vi "manual-move-general.vi"() -> ()   [LabVIEW 2011]
uses:
  <vilib>/userDefined/High Color/IMAQdx.ctl
panel:
  in  "stop":bool
  in  "Ring":u16(ring)=6 items=["*100TW Preamp Up", "*100TW Output Preamp2", "*100TW M0", "*100TW M8", "*100TW M9", "*100TW M10", "*100TW M13", "*100TW M14", "*100TW M20", "*100TW M22", "*100TW M23"]
  out "Names":string[](array[string])=["*100TW Preamp Up", "*100TW Output Preamp2", "*100TW M0", "*100TW M8", "*100TW M9", "*100TW M10", "*100TW M13", "*100TW M14", "*100TW M20", "*100TW M22", "*100TW M23"]
  in  "Step Size":u16=100
  in  "Manual Move":T1={"Down"=FALSE, "Up"=FALSE, "Right"=FALSE, "Left"=FALSE, "APulses X"=200, "APulses Y"=200, "StopButton"=FALSE}
  out "Last Move":string[](array[string])=["", "", "", "", "", "", "3:58:36 PM", "3:59:18 PM", ""]
  in  "CamConfigArray":T3(array[cluster])=[{"ID"=57.0, "Name"="*100TW Preamp Up", "DeviceID"={"Slot Connector"=11, "IP Adress"="192.168.10.34", "Port"=63420, "Type"="picodriver"}, "CorrectConfig Cluster"={"Detection Parameters"={"Contrast"=64, "Treshold"=64, "Max Intensity"=255, "Max Intensity%"=80, "Rx"=95, "Ry"=76, "R%"=70.0}, "Reverse"={"Reverse X"=FALSE, "Reverse Y"=TRUE}, "Target"={"X Target"=387.0, "Y Target"=278.0}, "Region of Interest"=[0, 0, 0, 0], "Correction Parameters"={"X"=30.0, "Y"=30.0, "Movement Type"=1}, "Acquisition Parameters"={"Brightness"=0.0, "Contrast"=0.0, "Saturation"=0.0, "White level"=0.0}, "Background Path"=path "", "Reference Path"=path "", "XCalibration"=[{-240.0, -16.0}, {-210.0, -14.0}, {-180.0, -11.0}, {-150.0, -10.0}, {-120.0, -8.0}, {-90.0, -5.0}, {-60.0, -3.0}, {-30.0, -2.0}, {0.0, -1.0}, {30.0, 0.0}, {60.0, 1.0}, {90.0, 2.0}, {120.0, 5.0}, {150.0, 7.0}, {180.0, 8.0}, {210.0, 9.0}, {240.0, 11.0}, {270.0, 14.0}], "YCalibration"=[{-240.0, 24.0}, {-210.0, 21.0}, {-180.0, 18.0}, {-150.0, 15.0}, {-120.0, 11.0}, {-90.0, 7.0}, {-60.0, 4.0}, {-30.0, 3.0}, {0.0, 1.0}, {30.0, -1.0}, {60.0, -3.0}, {90.0, -4.0}, {120.0, -6.0}, {150.0, -9.0}, {180.0, -12.0}, {210.0, -14.0}, {240.0, -16.0}, {270.0, -18.0}]}, "Ontrak Channel"=0, "IMAQdx Session 2"="cam2", "ImageServer"={"IPAddress"="234.5.6.8", "Port"=58451}}, {"ID"=59.0, "Name"="*100TW Output Preamp2", "DeviceID"={"Slot Connector"=14, "IP Adress"="192.168.10.34", "Port"=63420, "Type"="picodriver"}, "CorrectConfig Cluster"={"Detection Parameters"={"Contrast"=143, "Treshold"=143, "Max Intensity"=255, "Max Intensity%"=80, "Rx"=70, "Ry"=68, "R%"=50.0}, "Reverse"={"Reverse X"=FALSE, "Reverse Y"=FALSE}, "Target"={"X Target"=427.0, "Y Target"=302.0}, "Region of Interest"=[0, 0, 0, 0], "Correction Parameters"={"X"=40.0, "Y"=40.0, "Movement Type"=1}, "Acquisition Parameters"={"Brightness"=0.0, "Contrast"=0.0, "Saturation"=0.0, "White level"=0.0}, "Background Path"=path "", "Reference Path"=path "", "XCalibration"=[{-440.0, -10.0}, {-400.0, -10.0}, {-360.0, -10.0}, {-320.0, -9.0}, {-280.0, -8.0}, {-240.0, -7.0}, {-200.0, -6.0}, {-160.0, -4.0}, {-120.0, -4.0}, {-80.0, -3.0}, {-40.0, -1.0}, {0.0, -1.0}, {40.0, -0.0}, {80.0, 1.0}, {120.0, 2.0}, {160.0, 2.0}, {200.0, 4.0}, {240.0, 5.0}, {280.0, 5.0}, {320.0, 6.0}, {360.0, 7.0}, {400.0, 8.0}, {440.0, 7.0}], "YCalibration"=[{-440.0, 10.0}, {-400.0, 8.0}, {-360.0, 7.0}, {-320.0, 7.0}, {-280.0, 7.0}, {-240.0, 8.0}, {-200.0, 8.0}, {-160.0, 7.0}, {-120.0, 4.0}, {-80.0, 2.0}, {-40.0, 1.0}, {0.0, 1.0}, {40.0, -0.0}, {80.0, -1.0}, {120.0, -2.0}, {160.0, -2.0}, {200.0, -3.0}, {240.0, -3.0}, {280.0, -4.0}, {320.0, -4.0}, {360.0, -4.0}, {400.0, -6.0}, {440.0, -9.0}]}, "Ontrak Channel"=0, "IMAQdx Session 2"="cam2", "ImageServer"={"IPAddress"="234.5.6.8", "Port"=58453}}, {"ID"=60.0, "Name"="*100TW M0", "DeviceID"={"Slot Connector"=13, "IP Adress"="192.168.10.34", "Port"=63420, "Type"="picodriver"}, "CorrectConfig Cluster"={"Detection Parameters"={"Contrast"=58, "Treshold"=58, "Max Intensity"=255, "Max Intensity%"=80, "Rx"=45, "Ry"=42, "R%"=50.0}, "Reverse"={"Reverse X"=FALSE, "Reverse Y"=FALSE}, "Target"={"X Target"=373.0, "Y Target"=310.0}, "Region of Interest"=[0, 0, 0, 0], "Correction Parameters"={"X"=40.0, "Y"=40.0, "Movement Type"=1}, "Acquisition Parameters"={"Brightness"=0.0, "Contrast"=0.0, "Saturation"=0.0, "White level"=0.0}, "Background Path"=path "", "Reference Path"=path "", "XCalibration"=[{-560.0, -7.0}, {-520.0, -7.0}, {-480.0, -7.0}, {-440.0, -7.0}, {-400.0, -6.0}, {-360.0, -5.0}, {-320.0, -4.0}, {-280.0, -4.0}, {-240.0, -4.0}, {-200.0, -3.0}, {-160.0, -2.0}, {-120.0, -2.0}, {-80.0, -1.0}, {-40.0, -0.0}, {0.0, -0.0}, {40.0, -0.0}, {80.0, 0.0}, {120.0, 1.0}, {160.0, 1.0}, {200.0, 2.0}, {240.0, 2.0}, {280.0, 2.0}, {320.0, 2.0}, {360.0, 3.0}, {400.0, 4.0}, {440.0, 5.0}, {480.0, 5.0}, {520.0, 5.0}, {560.0, 5.0}], "YCalibration"=[{-560.0, 3.0}, {-520.0, 3.0}, {-480.0, 3.0}, {-440.0, 3.0}, {-400.0, 3.0}, {-360.0, 4.0}, {-320.0, 3.0}, {-280.0, 3.0}, {-240.0, 3.0}, {-200.0, 2.0}, {-160.0, 1.0}, {-120.0, 1.0}, {-80.0, 0.0}, {-40.0, -0.0}, {0.0, 0.0}, {40.0, 0.0}, {80.0, -0.0}, {120.0, -0.0}, {160.0, -1.0}, {200.0, -2.0}, {240.0, -3.0}, {280.0, -3.0}, {320.0, -3.0}, {360.0, -4.0}, {400.0, -4.0}, {440.0, -4.0}, {480.0, -4.0}, {520.0, -4.0}, {560.0, -4.0}]}, "Ontrak Channel"=0, "IMAQdx Session 2"="cam2", "ImageServer"={"IPAddress"="234.5.6.8", "Port"=58454}}, {"ID"=64.0, "Name"="*100TW M8", "DeviceID"={"Slot Connector"=24, "IP Adress"="192.168.10.34", "Port"=63420, "Type"="picodriver"}, "CorrectConfig Cluster"={"Detection Parameters"={"Contrast"=22, "Treshold"=22, "Max Intensity"=255, "Max Intensity%"=80, "Rx"=225, "Ry"=333, "R%"=50.0}, "Reverse"={"Reverse X"=TRUE, "Reverse Y"=FALSE}, "Target"={"X Target"=731.0, "Y Target"=501.0}, "Region of Interest"=[0, 0, 0, 0], "Correction Parameters"={"X"=50.0, "Y"=50.0, "Movement Type"=1}, "Acquisition Parameters"={"Brightness"=0.0, "Contrast"=0.0, "Saturation"=0.0, "White level"=0.0}, "Background Path"=path "", "Reference Path"=path "", "XCalibration"=[{-450.0, -14.0}, {-400.0, -12.0}, {-350.0, -10.0}, {-300.0, -9.0}, {-250.0, -8.0}, {-200.0, -6.0}, {-150.0, -5.0}, {-100.0, -3.0}, {-50.0, -2.0}, {0.0, -0.0}, {50.0, 1.0}, {100.0, 2.0}, {150.0, 4.0}, {200.0, 6.0}, {250.0, 8.0}, {300.0, 9.0}, {350.0, 11.0}, {400.0, 13.0}, {450.0, 16.0}], "YCalibration"=[{-450.0, 9.0}, {-400.0, 7.0}, {-350.0, 6.0}, {-300.0, 6.0}, {-250.0, 5.0}, {-200.0, 5.0}, {-150.0, 3.0}, {-100.0, 2.0}, {-50.0, 1.0}, {0.0, 0.0}, {50.0, -0.0}, {100.0, -1.0}, {150.0, -3.0}, {200.0, -4.0}, {250.0, -6.0}, {300.0, -7.0}, {350.0, -8.0}, {400.0, -9.0}, {450.0, -11.0}]}, "Ontrak Channel"=0, "IMAQdx Session 2"="cam2", "ImageServer"={"IPAddress"="234.5.6.8", "Port"=58450}}, {"ID"=55.0, "Name"="*100TW M9", "DeviceID"={"Slot Connector"=31, "IP Adress"="192.168.10.34", "Port"=63420, "Type"="picodriver"}, "CorrectConfig Cluster"={"Detection Parameters"={"Contrast"=5, "Treshold"=5, "Max Intensity"=255, "Max Intensity%"=80, "Rx"=400, "Ry"=300, "R%"=50.0}, "Reverse"={"Reverse X"=FALSE, "Reverse Y"=TRUE}, "Target"={"X Target"=771.0, "Y Target"=447.0}, "Region of Interest"=[0, 0, 0, 0], "Correction Parameters"={"X"=40.0, "Y"=40.0, "Movement Type"=1}, "Acquisition Parameters"={"Brightness"=0.0, "Contrast"=0.0, "Saturation"=0.0, "White level"=0.0}, "Background Path"=path "", "Reference Path"=path "", "XCalibration"=[{-320.0, -6.0}, {-280.0, -6.0}, {-240.0, -5.0}, {-200.0, -4.0}, {-160.0, -3.0}, {-120.0, -2.0}, {-80.0, -2.0}, {-40.0, -1.0}, {0.0, -0.0}, {40.0, 0.0}, {80.0, 1.0}, {120.0, 2.0}, {160.0, 2.0}, {200.0, 3.0}, {240.0, 4.0}, {280.0, 4.0}, {320.0, 5.0}, {360.0, 5.0}], "YCalibration"=[{-320.0, 4.0}, {-280.0, 4.0}, {-240.0, 3.0}, {-200.0, 3.0}, {-160.0, 3.0}, {-120.0, 2.0}, {-80.0, 1.0}, {-40.0, 1.0}, {0.0, 0.0}, {40.0, -0.0}, {80.0, -1.0}, {120.0, -1.0}, {160.0, -2.0}, {200.0, -3.0}, {240.0, -3.0}, {280.0, -3.0}, {320.0, -3.0}, {360.0, -3.0}]}, "Ontrak Channel"=0, "IMAQdx Session 2"="cam2", "ImageServer"={"IPAddress"="234.5.6.8", "Port"=58444}}, {"ID"=56.0, "Name"="*100TW M10", "DeviceID"={"Slot Connector"=32, "IP Adress"="192.168.10.34", "Port"=63420, "Type"="picodriver"}, "CorrectConfig Cluster"={"Detection Parameters"={"Contrast"=30, "Treshold"=30, "Max Intensity"=255, "Max Intensity%"=80, "Rx"=350, "Ry"=166, "R%"=50.0}, "Reverse"={"Reverse X"=FALSE, "Reverse Y"=TRUE}, "Target"={"X Target"=290.0, "Y Target"=222.0}, "Region of Interest"=[0, 0, 0, 0], "Correction Parameters"={"X"=30.0, "Y"=30.0, "Movement Type"=1}, "Acquisition Parameters"={"Brightness"=0.0, "Contrast"=0.0, "Saturation"=0.0, "White level"=0.0}, "Background Path"=path "", "Reference Path"=path "", "XCalibration"=[{-480.0, -20.0}, {-450.0, -18.0}, {-420.0, -17.0}, {-390.0, -16.0}, {-360.0, -15.0}, {-330.0, -14.0}, {-300.0, -13.0}, {-270.0, -12.0}, {-240.0, -11.0}, {-210.0, -9.0}, {-180.0, -8.0}, {-150.0, -6.0}, {-120.0, -5.0}, {-90.0, -4.0}, {-60.0, -3.0}, {-30.0, -2.0}, {0.0, -1.0}, {30.0, 1.0}, {60.0, 2.0}, {90.0, 3.0}, {120.0, 3.0}, {150.0, 4.0}, {180.0, 5.0}, {210.0, 6.0}, {240.0, 8.0}, {270.0, 9.0}, {300.0, 10.0}, {330.0, 11.0}, {360.0, 12.0}, {390.0, 12.0}, {420.0, 13.0}, {450.0, 14.0}, {480.0, 15.0}, {510.0, 16.0}], "YCalibration"=[{-480.0, 9.0}, {-450.0, 9.0}, {-420.0, 8.0}, {-390.0, 7.0}, {-360.0, 6.0}, {-330.0, 6.0}, {-300.0, 5.0}, {-270.0, 5.0}, {-240.0, 4.0}, {-210.0, 4.0}, {-180.0, 4.0}, {-150.0, 3.0}, {-120.0, 2.0}, {-90.0, 2.0}, {-60.0, 1.0}, {-30.0, 0.0}, {0.0, 0.0}, {30.0, -0.0}, {60.0, -0.0}, {90.0, -1.0}, {120.0, -2.0}, {150.0, -2.0}, {180.0, -3.0}, {210.0, -4.0}, {240.0, -4.0}, {270.0, -4.0}, {300.0, -5.0}, {330.0, -6.0}, {360.0, -6.0}, {390.0, -7.0}, {420.0, -8.0}, {450.0, -9.0}, {480.0, -9.0}, {510.0, -10.0}]}, "Ontrak Channel"=0, "IMAQdx Session 2"="cam2", "ImageServer"={"IPAddress"="234.5.6.8", "Port"=58445}}, {"ID"=65.0, "Name"="*100TW M13", "DeviceID"={"Slot Connector"=33, "IP Adress"="192.168.10.34", "Port"=63420, "Type"="picodriver"}, "CorrectConfig Cluster"={"Detection Parameters"={"Contrast"=0, "Treshold"=0, "Max Intensity"=0, "Max Intensity%"=0, "Rx"=0, "Ry"=0, "R%"=0.0}, "Reverse"={"Reverse X"=FALSE, "Reverse Y"=FALSE}, "Target"={"X Target"=0.0, "Y Target"=0.0}, "Region of Interest"=[0, 0, 0, 0], "Correction Parameters"={"X"=0.0, "Y"=0.0, "Movement Type"=0}, "Acquisition Parameters"={"Brightness"=0.0, "Contrast"=0.0, "Saturation"=0.0, "White level"=0.0}, "Background Path"=path "", "Reference Path"=path "", "XCalibration"=[], "YCalibration"=[]}, "Ontrak Channel"=0, "IMAQdx Session 2"="cam2", "ImageServer"={"IPAddress"="127.0.0.1", "Port"=3500}}, {"ID"=65.0, "Name"="*100TW M14", "DeviceID"={"Slot Connector"=11, "IP Adress"="192.168.10.73", "Port"=63430, "Type"="picodriver"}, "CorrectConfig Cluster"={"Detection Parameters"={"Contrast"=0, "Treshold"=0, "Max Intensity"=0, "Max Intensity%"=0, "Rx"=0, "Ry"=0, "R%"=0.0}, "Reverse"={"Reverse X"=FALSE, "Reverse Y"=FALSE}, "Target"={"X Target"=0.0, "Y Target"=0.0}, "Region of Interest"=[0, 0, 0, 0], "Correction Parameters"={"X"=0.0, "Y"=0.0, "Movement Type"=0}, "Acquisition Parameters"={"Brightness"=0.0, "Contrast"=0.0, "Saturation"=0.0, "White level"=0.0}, "Background Path"=path "", "Reference Path"=path "", "XCalibration"=[], "YCalibration"=[]}, "Ontrak Channel"=0, "IMAQdx Session 2"="cam2", "ImageServer"={"IPAddress"="127.0.0.1", "Port"=3500}}, {"ID"=0.0, "Name"="*100TW M20", "DeviceID"={"Slot Connector"=1, "IP Adress"="192.168.10.184", "Port"=63430, "Type"="picodriver"}, "CorrectConfig Cluster"={"Detection Parameters"={"Contrast"=73, "Treshold"=73, "Max Intensity"=255, "Max Intensity%"=80, "Rx"=100, "Ry"=95, "R%"=95.0}, "Reverse"={"Reverse X"=TRUE, "Reverse Y"=TRUE}, "Target"={"X Target"=512.0, "Y Target"=384.0}, "Region of Interest"=[0, 0, 0, 0], "Correction Parameters"={"X"=10.0, "Y"=10.0, "Movement Type"=0}, "Acquisition Parameters"={"Brightness"=0.0, "Contrast"=0.0, "Saturation"=0.0, "White level"=0.0}, "Background Path"=path "", "Reference Path"=path "", "XCalibration"=[{-700.0, -90.0}, {-600.0, -65.0}, {-500.0, -44.0}, {-400.0, -30.0}, {-300.0, -23.0}, {-200.0, -17.0}, {-100.0, -12.0}, {0.0, -6.0}, {100.0, -2.0}, {200.0, -0.0}, {300.0, 3.0}, {400.0, 9.0}, {500.0, 21.0}, {600.0, 41.0}, {700.0, 66.0}], "YCalibration"=[{-700.0, 147.0}, {-600.0, 130.0}, {-500.0, 115.0}, {-400.0, 100.0}, {-300.0, 81.0}, {-200.0, 52.0}, {-100.0, 23.0}, {0.0, 4.0}, {100.0, -11.0}, {200.0, -36.0}, {300.0, -66.0}, {400.0, -86.0}, {500.0, -100.0}, {600.0, -114.0}, {700.0, -130.0}]}, "Ontrak Channel"=0, "IMAQdx Session 2"="cam2", "ImageServer"={"IPAddress"="234.5.6.8", "Port"=58443}}, {"ID"=12.0, "Name"="*100TW M22", "DeviceID"={"Slot Connector"=3, "IP Adress"="192.168.10.184", "Port"=63430, "Type"="picodriver"}, "CorrectConfig Cluster"={"Detection Parameters"={"Contrast"=50, "Treshold"=10, "Max Intensity"=255, "Max Intensity%"=80, "Rx"=60, "Ry"=60, "R%"=90.0}, "Reverse"={"Reverse X"=FALSE, "Reverse Y"=TRUE}, "Target"={"X Target"=306.0, "Y Target"=222.0}, "Region of Interest"=[0, 0, 0, 0], "Correction Parameters"={"X"=1000.0, "Y"=1000.0, "Movement Type"=1}, "Acquisition Parameters"={"Brightness"=0.0, "Contrast"=0.0, "Saturation"=0.0, "White level"=0.0}, "Background Path"=path "", "Reference Path"=path "", "XCalibration"=[{0.0, 0.0}, {1000.0, -42.0}], "YCalibration"=[{0.0, 0.0}, {1000.0, 183.0}]}, "Ontrak Channel"=0, "IMAQdx Session 2"="cam2", "ImageServer"={"IPAddress"="234.5.6.8", "Port"=58446}}, {"ID"=12.0, "Name"="*100TW M23", "DeviceID"={"Slot Connector"=4, "IP Adress"="192.168.10.184", "Port"=63430, "Type"="picodriver"}, "CorrectConfig Cluster"={"Detection Parameters"={"Contrast"=0, "Treshold"=0, "Max Intensity"=255, "Max Intensity%"=80, "Rx"=-15, "Ry"=-15, "R%"=50.0}, "Reverse"={"Reverse X"=FALSE, "Reverse Y"=TRUE}, "Target"={"X Target"=303.0, "Y Target"=342.0}, "Region of Interest"=[0, 0, 0, 0], "Correction Parameters"={"X"=0.0, "Y"=0.0, "Movement Type"=0}, "Acquisition Parameters"={"Brightness"=0.0, "Contrast"=0.0, "Saturation"=0.0, "White level"=0.0}, "Background Path"=path "", "Reference Path"=path "", "XCalibration"=[], "YCalibration"=[]}, "Ontrak Channel"=0, "IMAQdx Session 2"="cam2", "ImageServer"={"IPAddress"="234.5.6.8", "Port"=58448}}] {"CorrectConfig Cluster"."Acquisition Parameters"."White level" scale=0.3..1.26 scale format="%#_2f"; "CorrectConfig Cluster"."Acquisition Parameters"."Saturation" scale=0.5..1.5 scale format="%#_3f"; "CorrectConfig Cluster"."Acquisition Parameters"."Contrast" scale=0.4..1.5 scale format="%#_3f"; "CorrectConfig Cluster"."Acquisition Parameters"."Brightness" scale=-50.0..50.0 scale format="%#_2f"; "CorrectConfig Cluster"."Correction Parameters"."Movement Type" items=["Step", "Proportionnal"]; "CorrectConfig Cluster"."Target"."X Target" format="%#_5g"; "CorrectConfig Cluster"."Target"."Y Target" format="%#_5g"; "CorrectConfig Cluster"."Detection Parameters"."Max Intensity%" max=100 step=1}
  out "TCPconnecCmd":bool=TRUE
  out "ConnectArray":T4(array[cluster])=[{"IPaddress"="192.168.10.184", "Port"=63430, "connection ID"=refnum, "TCP error"={"status"=FALSE, "code"=0, "source"=""}}]
  out "Status":string="OK"
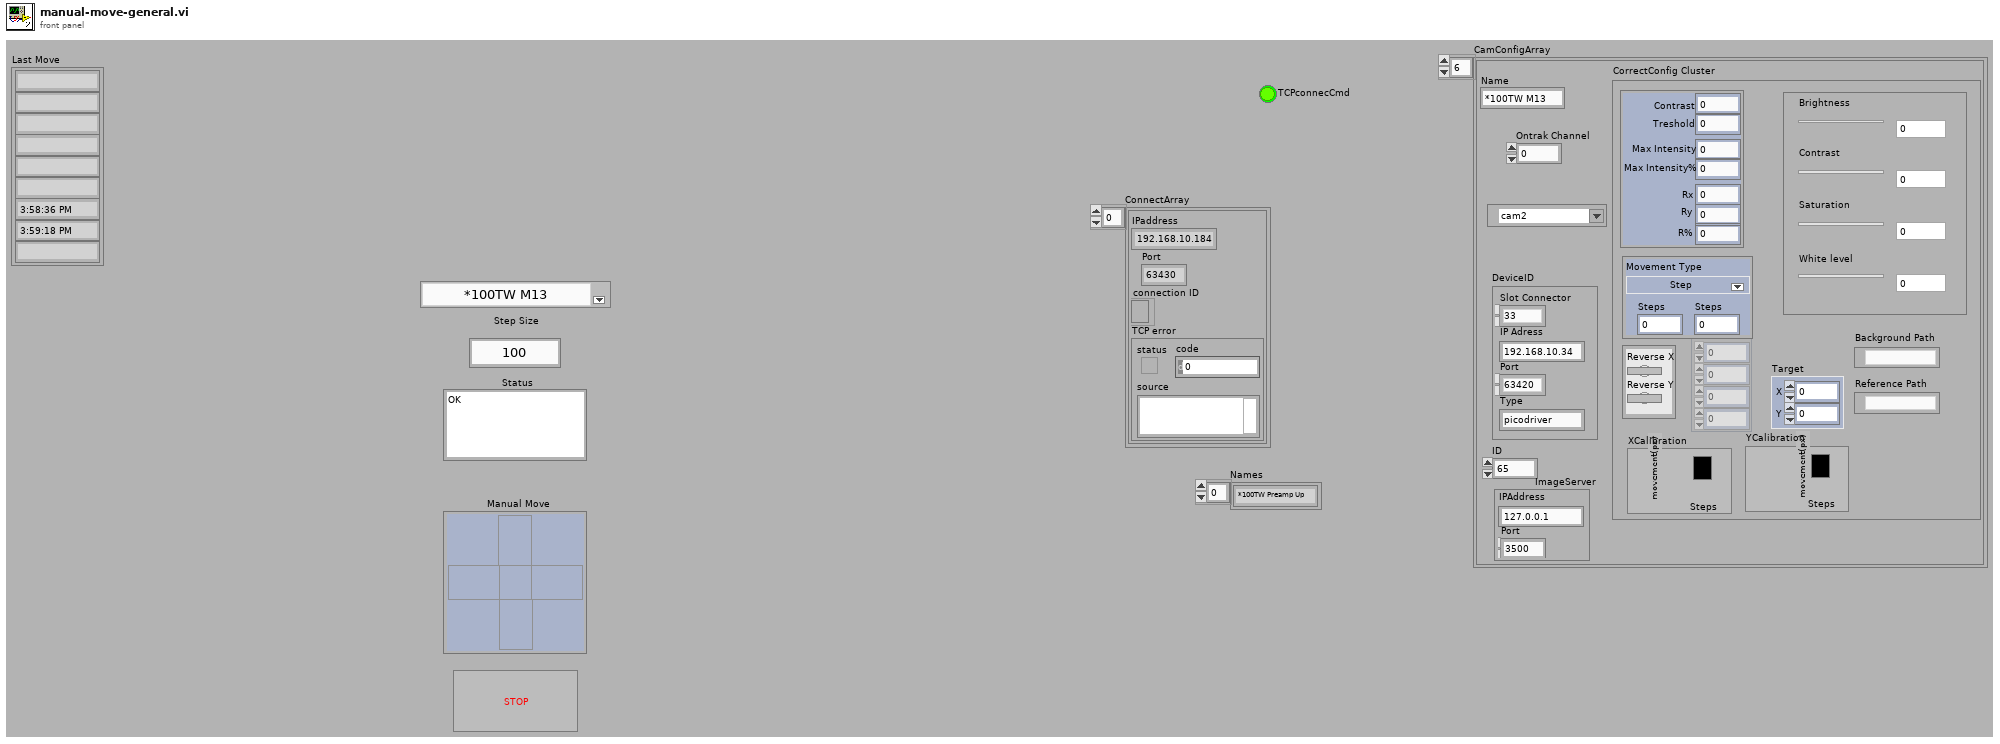
[diagram p1: front panel]
types:
  T1 = cluster{"Down":bool, "Up":bool, "Right":bool, "Left":bool, "APulses X":u16, "APulses Y":u16, "StopButton":bool}
  T2 = typedef "IMAQdx.ctl" = refnum<k21>
  T3 = cluster{"ID":dbl, "Name":string, "DeviceID":cluster{"Slot Connector":i32, "IP Adress":string, "Port":i32, "Type":string}, "CorrectConfig Cluster":cluster{"Detection Parameters":cluster{"Contrast":i32, "Treshold":u8, "Max Intensity":i32, "Max Intensity%":u8, "Rx":i32, "Ry":i32, "R%":sgl}, "Reverse":cluster{"Reverse X":bool, "Reverse Y":bool}, "Target":cluster{"X Target":sgl, "Y Target":sgl}, "Region of Interest":i32[], "Correction Parameters":cluster{"X":sgl, "Y":sgl, "Movement Type":u16}, "Acquisition Parameters":cluster{"Brightness":dbl, "Contrast":dbl, "Saturation":dbl, "White level":dbl}, "Background Path":path, "Reference Path":path, "XCalibration":cluster{dbl, dbl}[], "YCalibration":cluster{dbl, dbl}[]}, "Ontrak Channel":i16, "IMAQdx Session 2":T2, "ImageServer":cluster{"IPAddress":string, "Port":i32}}[]
  T4 = cluster{"IPaddress":string, "Port":i32, "connection ID":refnum<k5>, "TCP error":errorcluster}[]
  T5 = cluster{"ID":dbl, "Name":string, "DeviceID":cluster{"Slot Connector":i32, "IP Adress":string, "Port":i32, "Type":string}, "CorrectConfig Cluster":cluster{"Detection Parameters":cluster{"Contrast":i32, "Treshold":u8, "Max Intensity":i32, "Max Intensity%":u8, "Rx":i32, "Ry":i32, "R%":sgl}, "Reverse":cluster{"Reverse X":bool, "Reverse Y":bool}, "Target":cluster{"X Target":sgl, "Y Target":sgl}, "Region of Interest":i32[], "Correction Parameters":cluster{"X":sgl, "Y":sgl, "Movement Type":u16}, "Acquisition Parameters":cluster{"Brightness":dbl, "Contrast":dbl, "Saturation":dbl, "White level":dbl}, "Background Path":path, "Reference Path":path, "XCalibration":cluster{dbl, dbl}[], "YCalibration":cluster{dbl, dbl}[]}, "Ontrak Channel":i16, "IMAQdx Session 2":T2, "ImageServer":cluster{"IPAddress":string, "Port":i32}}
  T6 = cluster{"Down":bool, "Up":bool, "Right":bool, "Left":bool, "APulses X":u16, "APulses Y":u16, "StopButton":bool}[]
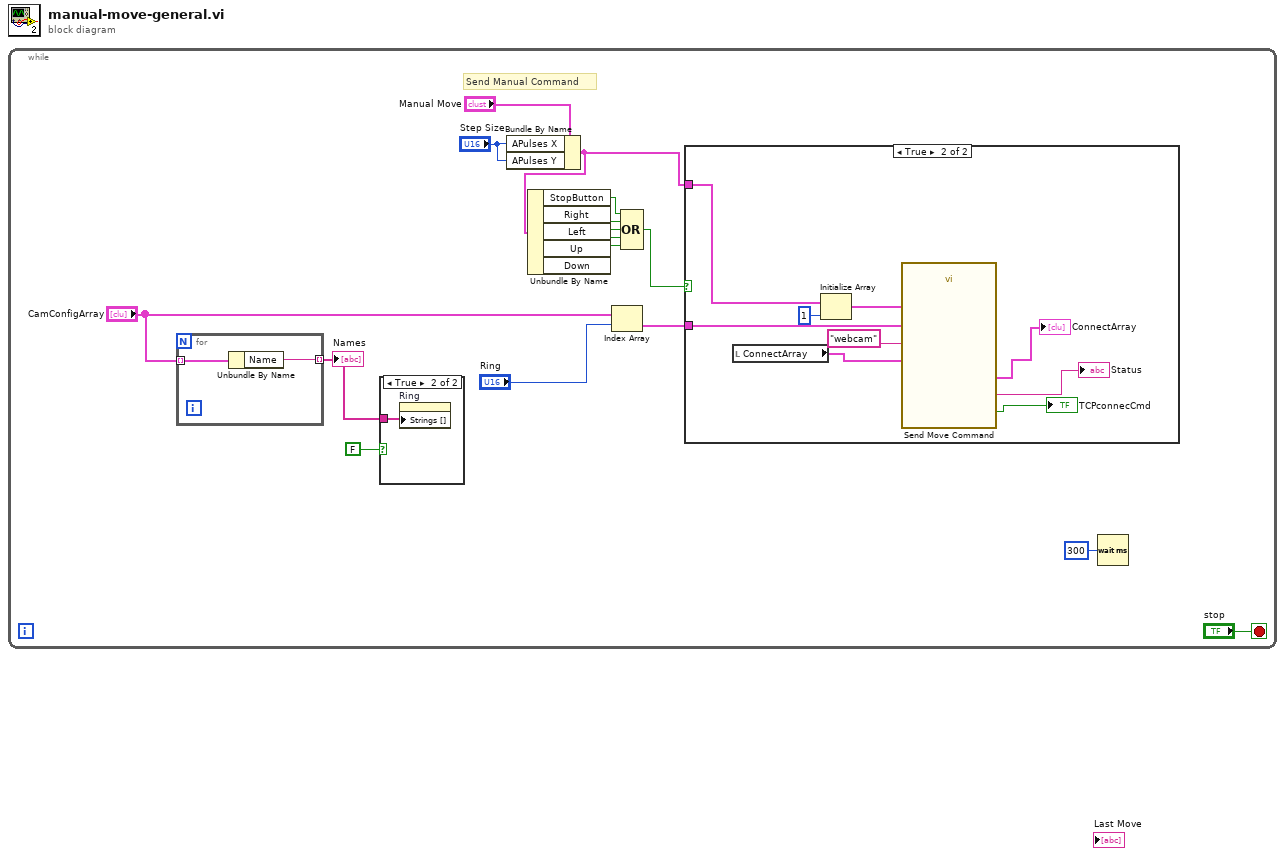
[diagram p0: block diagram]
diagram:
  n1 = while {
    stop <- "stop" stop-if-true
    # "Send Manual Command"
    n2 = for {
      tunnel: "CamConfigArray" -> [w19] mode=indexing
      tunnel: [w18] -> w5 mode=indexing
      n3 = Unbundle By Name(w19) -> ("Name"=w18:string)
    }
    "Names" <- w5
    n4 = case shown="True" FALSE {
      tunnel: w5 -> [_ w17]
      frame False {
      }
      frame True {
        n5 = property on="Ring" class="Ring (strict)"("Strings []"=w17) -> ()  [unwired: 2 in, 2 out]
      }
    }
    n6 = Bundle By Name(cluster="Manual Move", "APulses X"="Step Size", "APulses Y"="Step Size") -> (w8:T1)
    n7 = Unbundle By Name(w8) -> ("StopButton"=w12:bool, "Right"=w16:bool, "Left"=w15:bool, "Up"=w14:bool, "Down"=w13:bool)
    n8 = Index Array(array="CamConfigArray", index="Ring") -> (element=w11:T5)
    n9 = Compound Arithmetic op=OR(w12, w16, w15, w14, w13) -> (w7:bool)
    n10 = case shown="True" w7 {
      tunnel: w11 -> [_ w28]
      tunnel: w8 -> [_ w27]
      frame False {
      }
      frame True {
        n11 = local read "ConnectArray"() -> (w24:T4)
        n12 = Initialize Array(w27, 1 ("dimension size")) -> (w26:T6)
        n13 = call "Send Move Command.vi"("ConnectArray IN"=w24, "client name"="webcam", "CamConfig"=w28, "Move XY"=w26) -> ("ConnectArray Out"=→"ConnectArray":T4, "TCPconnecCmd"=→"TCPconnecCmd":bool, "status"=→"Status":string)
      }
    }
    n14 = Wait (ms)(milliseconds to wait=u32 300) -> ()  [unwired: 1 out]
  }
